vi "WLAN_be_EVM_SG_RS.vi"(5 "Function_SG":T1, 7 "setPower":i32, 8 "error in":errorcluster, 11 "VISA IN":refnum<visa-resource-name>="TCPIP::192.168.88.12::hislip0::INSTR") -> (0 "error out":errorcluster, 3 "IDN":string)   [LabVIEW 2023, in "R_S.lvlib"]
uses:
  R_S.lvlib
  CTL/LitePoint_EVM_SG.ctl
panel:
  # "TCPIP::192.168.88.12::hislip0::INSTR"
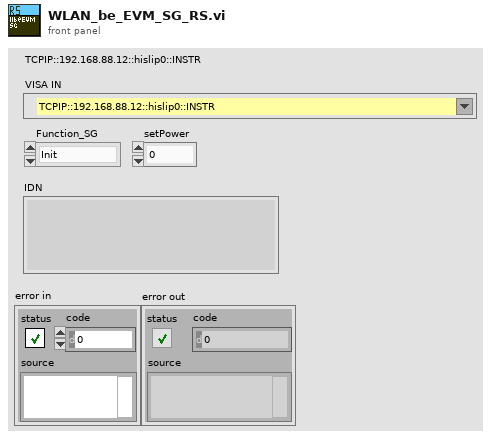
[diagram p1: front panel]
types:
  T1 = typedef "LitePoint_EVM_SG.ctl" = enum16{"Init", "Close", "set_SG", "AdjustLevel", "byPass", "RF_ON", "RF_OFF"}
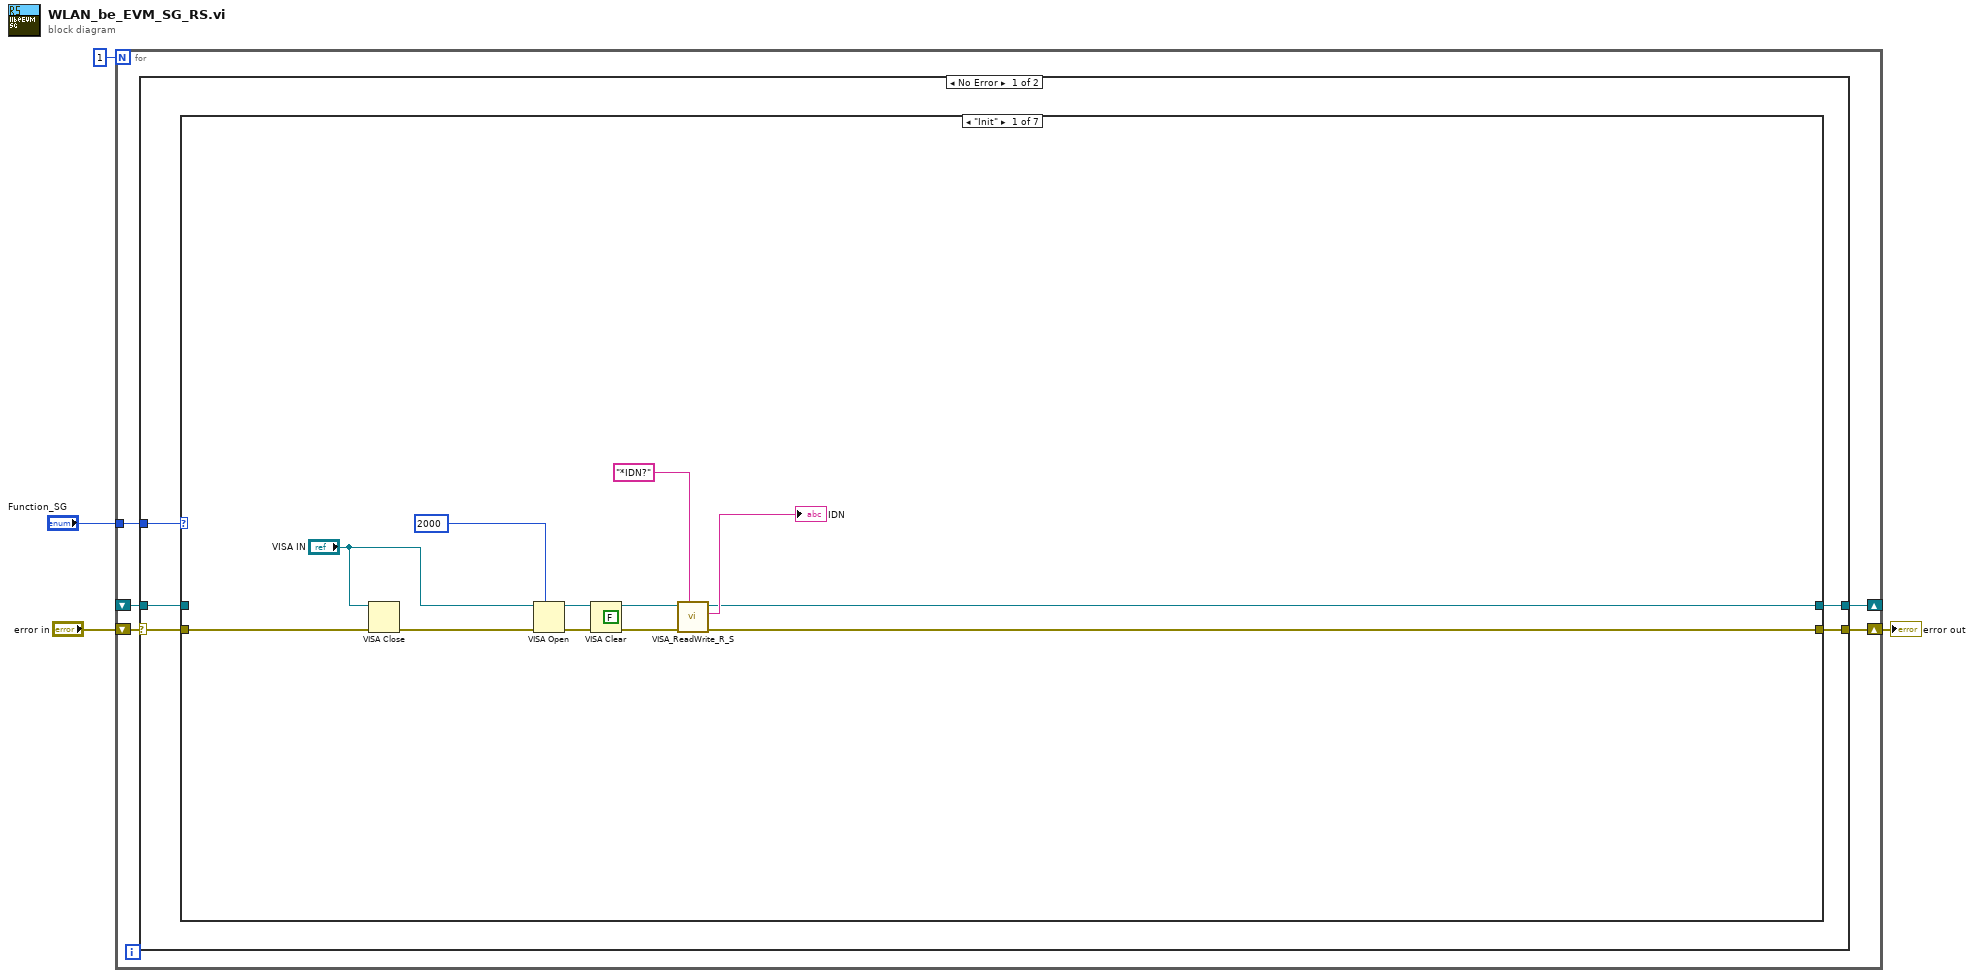
[diagram p0: block diagram]
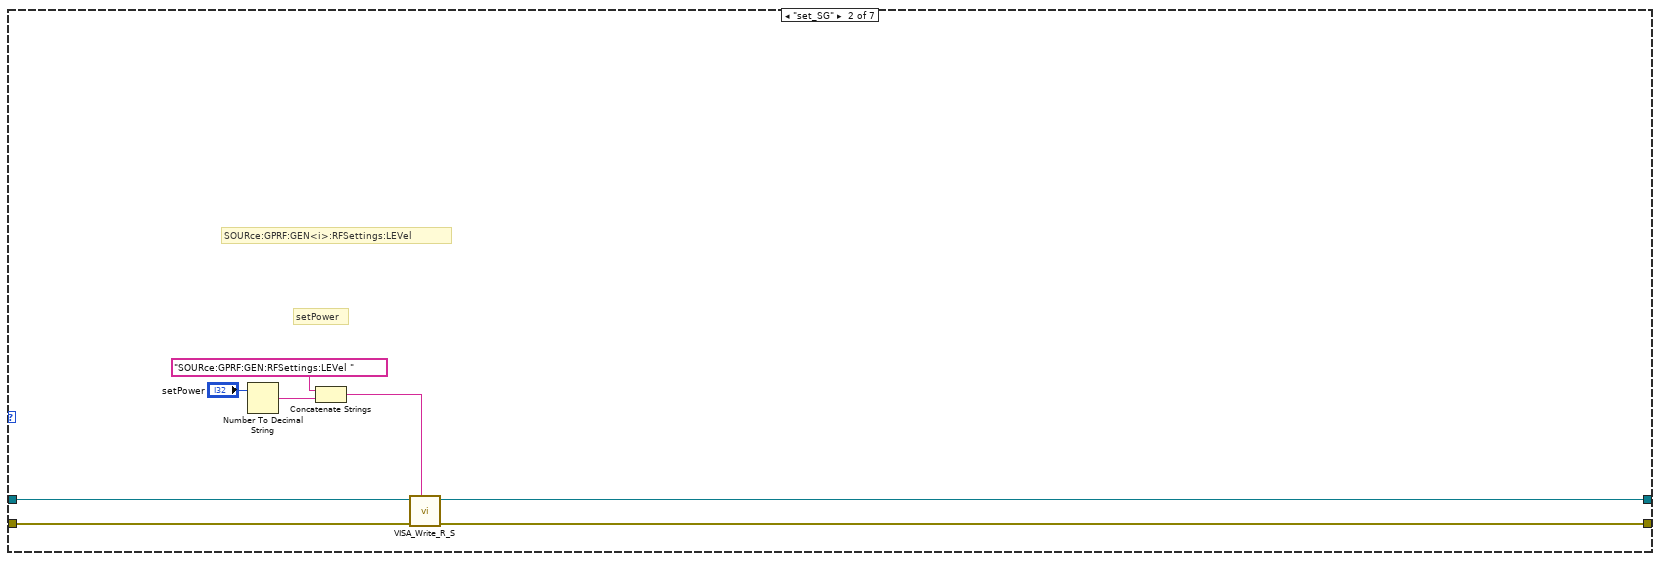
[diagram p2: hidden frame]
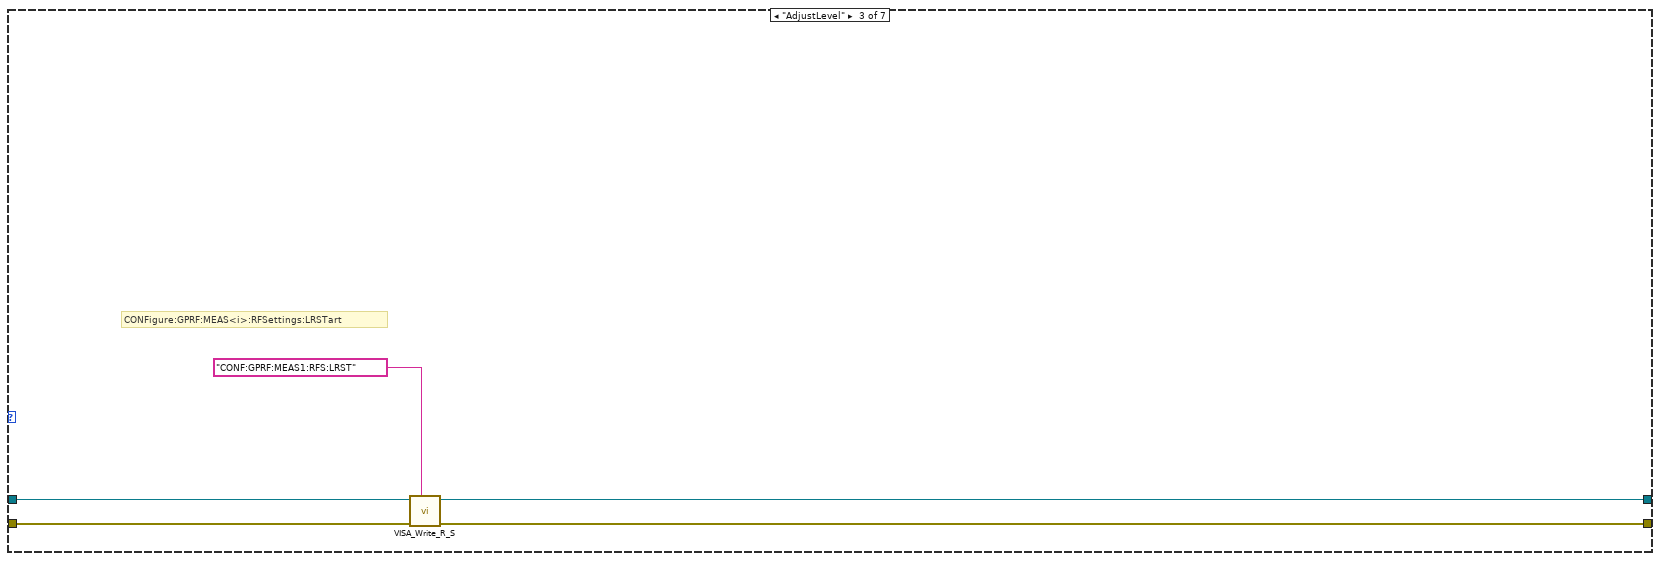
[diagram p3: hidden frame]
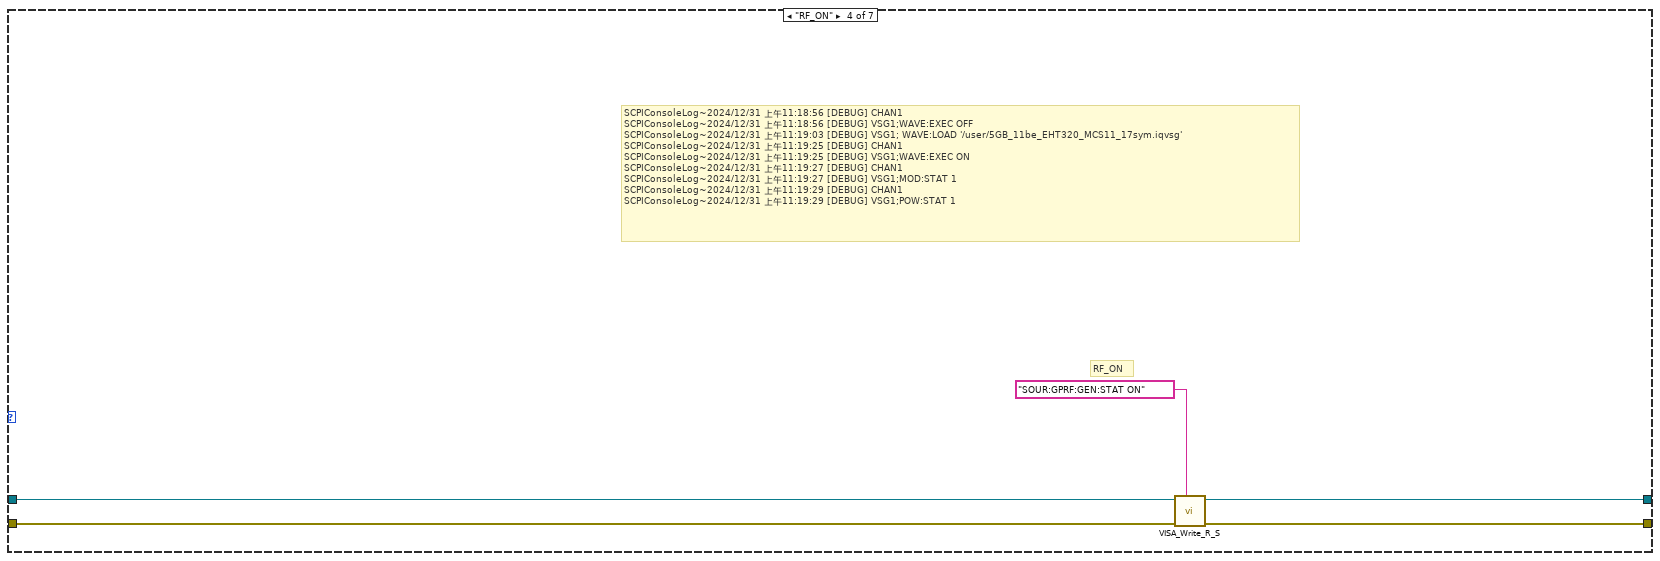
[diagram p4: hidden frame]
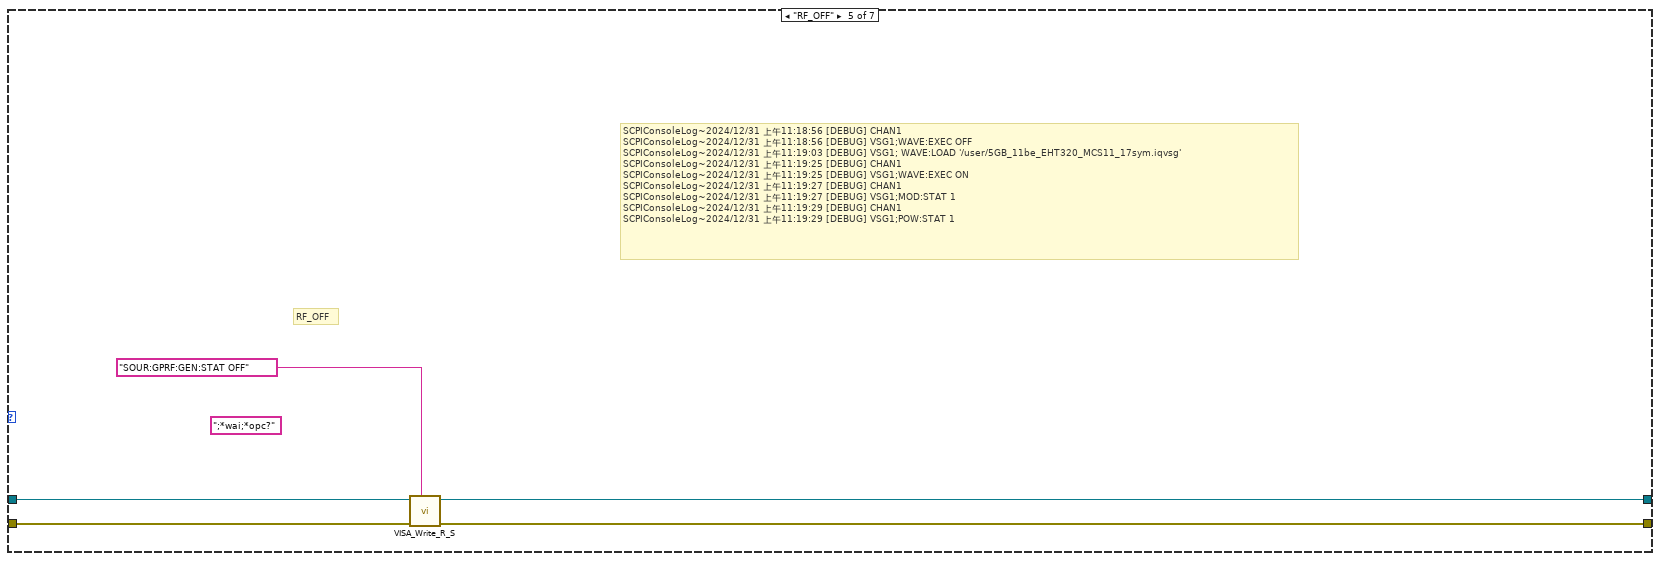
[diagram p5: hidden frame]
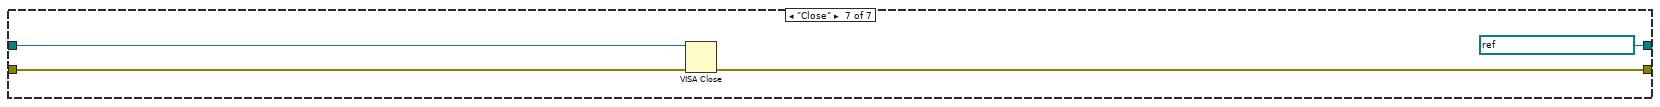
[diagram p7: hidden frame]
diagram:
  n1 = for {
    N: 1 -> [_]
    tunnel: "Function_SG" -> [w7]
    shift-right: [w8] -> w3
    shift-left: "error in" -> [w9]
    shift-right: [w5] -> _
    shift-left: _ -> [w6]
    n2 = case shown="No Error" w9 {
      selector: w9 -> [w13 w57]
      tunnel: [w12 w57] -> w8
      tunnel: w7 -> [w14 _]
      tunnel: w6 -> [w11 w56]
      tunnel: [w10 w56] -> w5
      frame No Error {
        n3 = case shown="\"Init\"" w14 {
          tunnel: [w22 w27 w36 w43 w46 w51 w55] -> w12
          tunnel: w13 -> [w17 w30 w38 w40 w48 w51 w54]
          tunnel: w11 -> [_ w31 w39 w41 w49 w50 w53]
          tunnel: [w18 w28 w37 w44 w47 w50 refnum<visa-resource-name> refnum ("VISA out")] -> w10
          frame "Init" {
            (unwired) FALSE ("duplicate session (F)")
            n4 = VISA Close(VISA resource name="VISA IN", error in (no error)=w17) -> (error out=w16:errorcluster)
            n5 = VISA Open(timeout (0)=u32 2000 ("VISA Open timeout (0)"), error in (no error)=w16, VISA resource name="VISA IN") -> (VISA resource name=w24:refnum<visa-resource-name>, error out=w25:errorcluster)  [unwired: 2 in]
            n6 = VISA Clear(VISA resource name=w24, error in (no error)=w25) -> (VISA resource name out=w21:refnum<visa-resource-name>, error out=w23:errorcluster)
            n7 = call "VISA_ReadWrite_R_S.vi"("VISA_CMD"="*IDN?", "error in"=w23, "VISA in"=w21) -> ("error out"=w22:errorcluster, "Response"=→"IDN":string, "VISA out"=w18:refnum<visa-resource-name>)  [unwired: 6 in]
          }
          frame "set_SG" {
            # "SOURce:GPRF:GEN<i>:RFSettings:LEVel"
            # "setPower"
            n8 = Number To Decimal String(number="setPower") -> (decimal integer string=w34:string)  [unwired: 1 in]
            n9 = Concatenate Strings("SOURce:GPRF:GEN:RFSettings:LEVel " ("write buffer"), w34) -> (w29:string)
            n10 = call "VISA_Write_R_S.vi"("VISA CMD"=w29, "error in"=w30, "VISA in"=w31) -> ("error out"=w27:errorcluster, "VISA out"=w28:refnum<visa-resource-name>)  [unwired: 7 in]
          }
          frame "AdjustLevel" {
            # "CONFigure:GPRF:MEAS<i>:RFSettings:LRSTart"
            n11 = call "VISA_Write_R_S.vi"("VISA CMD"="CONF:GPRF:MEAS1:RFS:LRST" ("write buffer"), "error in"=w38, "VISA in"=w39) -> ("error out"=w36:errorcluster, "VISA out"=w37:refnum<visa-resource-name>)  [unwired: 7 in]
          }
          frame "RF_ON" {
            # "SCPIConsoleLog~2024/12/31 上午11:18:56 [DEBUG] CHAN1\nSCPIConsoleLog~2024/12/31 上午11:18:56 [DEBUG] VSG1;WAVE:EXEC OFF\nSCPIConsoleLog~2024/12/31 上午11:19:03 [DEBUG] VSG1; WAVE:LOAD '/user/5GB_11be_EHT320_MCS11_17sym.iqvsg'\nSCPIConsoleLog~2024/12/31 上午11:19:25 [DEBUG] CHAN1\nSCPIConsoleLog~2024/12/31 上午11:19:25 [DEBUG] VSG1;WAVE:EXEC ON\nSCPIConsoleLog~2024/12/31 上午11:19:27 [DEBUG] CHAN1\nSCPIConsoleLog~2024/12/31 上午11:19:27 [DEBUG] VSG1;MOD:STAT 1\nSCPIConsoleLog~2024/12/31 上午11:19:29 [DEBUG] CHAN1\nSCPIConsoleLog~2024/12/31 上午11:19:29 [DEBUG] VSG1;POW:STAT 1"
            # "RF_ON"
            n12 = call "VISA_Write_R_S.vi"("VISA CMD"="SOUR:GPRF:GEN:STAT ON" ("write buffer"), "error in"=w40, "VISA in"=w41) -> ("error out"=w43:errorcluster, "VISA out"=w44:refnum<visa-resource-name>)  [unwired: 7 in]
          }
          frame "RF_OFF" {
            (unwired) ";*wai;*opc?" ("write buffer")
            # "SCPIConsoleLog~2024/12/31 上午11:18:56 [DEBUG] CHAN1\nSCPIConsoleLog~2024/12/31 上午11:18:56 [DEBUG] VSG1;WAVE:EXEC OFF\nSCPIConsoleLog~2024/12/31 上午11:19:03 [DEBUG] VSG1; WAVE:LOAD '/user/5GB_11be_EHT320_MCS11_17sym.iqvsg'\nSCPIConsoleLog~2024/12/31 上午11:19:25 [DEBUG] CHAN1\nSCPIConsoleLog~2024/12/31 上午11:19:25 [DEBUG] VSG1;WAVE:EXEC ON\nSCPIConsoleLog~2024/12/31 上午11:19:27 [DEBUG] CHAN1\nSCPIConsoleLog~2024/12/31 上午11:19:27 [DEBUG] VSG1;MOD:STAT 1\nSCPIConsoleLog~2024/12/31 上午11:19:29 [DEBUG] CHAN1\nSCPIConsoleLog~2024/12/31 上午11:19:29 [DEBUG] VSG1;POW:STAT 1"
            # "RF_OFF"
            n13 = call "VISA_Write_R_S.vi"("VISA CMD"="SOUR:GPRF:GEN:STAT OFF" ("write buffer"), "error in"=w48, "VISA in"=w49) -> ("error out"=w46:errorcluster, "VISA out"=w47:refnum<visa-resource-name>)  [unwired: 7 in]
          }
          frame "byPass", Default {
          }
          frame "Close" {
            n14 = VISA Close(VISA resource name=w53, error in (no error)=w54) -> (error out=w55:errorcluster)
          }
        }
      }
      frame Error {
      }
    }
  }
  "error out" <- w3
